vi "CCD_GPIB_Clear.vi"(2 "#device clearings":i32=3, 3 "error in":errorcluster, 4 "Device Clear?":bool=TRUE, 5 "GPIB Address":i16=1) -> (0 "error out":errorcluster)   [LabVIEW 2024]
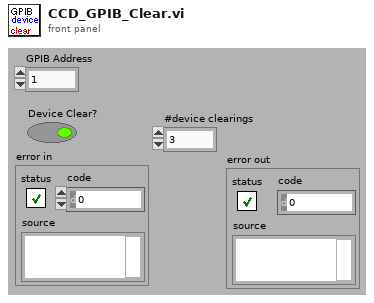
[diagram p1: front panel]
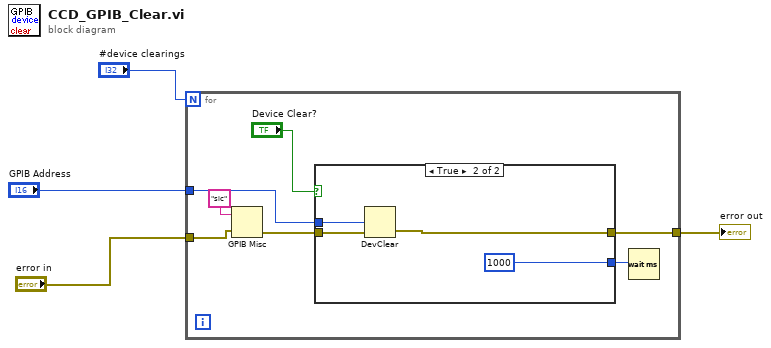
[diagram p0: block diagram]
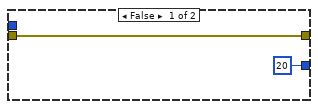
[diagram p2: hidden frame]
diagram:
  n1 = for {
    N: "#device clearings" -> [_]
    tunnel: [w9] -> w4
    tunnel: "GPIB Address" -> [w8]
    tunnel: "error in" -> [w7]
    n2 = GPIB Misc(0:"sic", 1:w7) -> (4:w10:errorcluster)  [unwired: 2 out]
    n3 = case shown="True" "Device Clear?" {
      tunnel: w10 -> [w13 w17]
      tunnel: [w13 w16] -> w9
      tunnel: w8 -> [_ w15]
      tunnel: [u32 20 ("milliseconds to wait") u32 1000 ("milliseconds to wait")] -> w5
      frame False {
      }
      frame True {
        n4 = DevClear(2:w17, 3:w15) -> (0:w16:errorcluster)  [unwired: 1 in, 1 out]
      }
    }
    n5 = Wait (ms)(milliseconds to wait=w5) -> ()  [unwired: 1 out]
  }
  "error out" <- w4
